vi "CalcDist2Circle.vi"(2 "Horizontal pixels from center":dbl, 3 "Height of circle":dbl=10.0) -> (0 "Distance sideways":dbl, 1 "Distance":dbl)   [LabVIEW 2009]
panel:
  out "Angle to circle":dbl
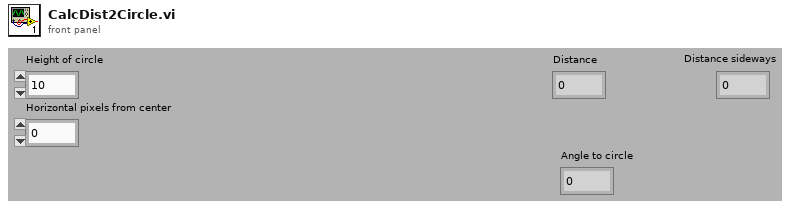
[diagram p1: front panel]
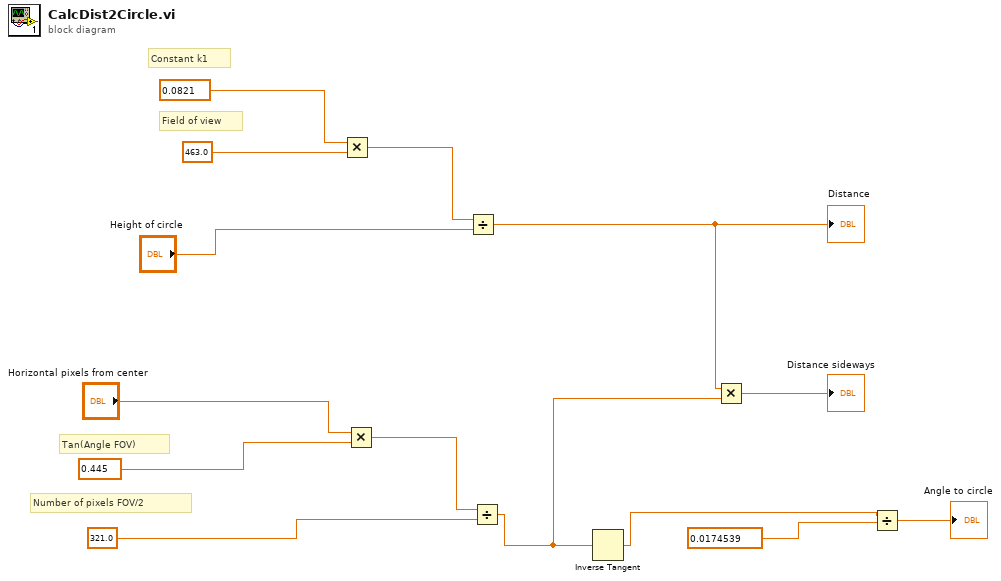
[diagram p0: block diagram]
diagram:
  # "Number of pixels FOV/2"
  # "Tan(Angle FOV)"
  # "Constant k1"
  # "Field of view"
  n1 = Multiply(x=0.0821, y=463.0) -> (x*y=w13:dbl)
  n2 = Multiply(x="Horizontal pixels from center", y=0.445) -> (x*y=w11:dbl)
  n3 = Divide(x=w13, y="Height of circle") -> (x/y=w7:dbl)
  "Distance" <- w7
  n4 = Divide(x=w11, y=321.0) -> (x/y=w6:dbl)
  n5 = Inverse Tangent(1:w6) -> (0:w3:dbl)
  n6 = Multiply(x=w7, y=w6) -> (x*y=→"Distance sideways":dbl)
  n7 = Divide(x=w3, y=0.0174539) -> (x/y=→"Angle to circle":dbl)
